vi "Validate Section ID.vi"(6 "Name":string, 8 "error in (no error)":errorcluster, 11 "Ref ID in":T1 format="%.0x") -> (0 "error out":errorcluster, 3 "Ref ID out":T1 format="%.0x")   [LabVIEW 2017, in "SLSC Switch Scripting.lvlib"]
uses:
  <vilib>/NI Veristand/Custom Device API/Custom Device Item Ref.ctl
  NationalInstruments.VeriStand.SystemDefinitionAPI
  SLSC Switch Scripting.lvlib
  <vilib>/NI VeriStand/Custom Device API/Custom Device API.lvlib
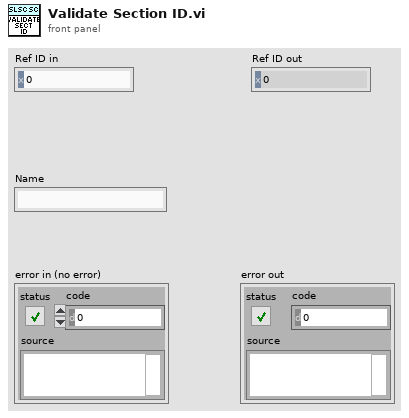
[diagram p1: front panel]
types:
  T1 = typedef "Custom Device API.lvlib/Custom Device Item Ref.ctl" = u64
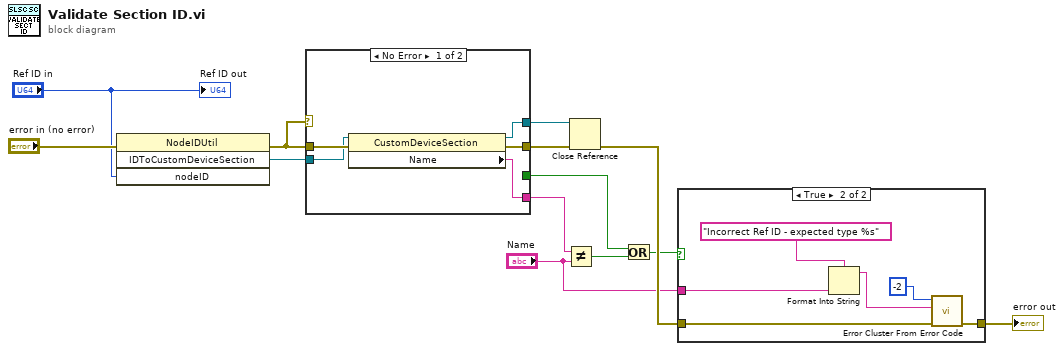
[diagram p0: block diagram]
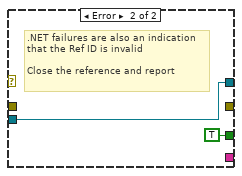
[diagram p2: hidden frame]
diagram:
  n1 = invoke class="NodeIDUtil" method="IDToCustomDeviceSection"(error in="error in (no error)", "nodeID"="Ref ID in") -> (error out=w4:errorcluster, "IDToCustomDeviceSection"=w10:refnum<k24>)  [unwired: 2 in, 2 out]
  n2 = case shown="No Error" w4 {
    tunnel: [w18 _] -> w13
    tunnel: [w17 _] -> w12
    tunnel: [w16 w20] -> w11
    tunnel: w4 -> [w15 _]
    tunnel: w10 -> [w14 w20]
    tunnel: [_ TRUE] -> w2
    frame No Error {
      n3 = property class="CustomDeviceSection"(reference=w14, error in=w15) -> (reference out=w16:refnum<k24>, error out=w17:errorcluster, "Name"=w18:string)
    }
    frame Error {
      # ".NET failures are also an indication\nthat the Ref ID is invalid\n\nClose the reference and report"
    }
  }
  n4 = Not Equal?(x=w13, y="Name") -> (x != y?=w1:bool)
  n5 = Close Reference(reference=w11, error in (no error)=w12) -> (error out=w8:errorcluster)
  n6 = Or(x=w2, y=w1) -> (x .or. y?=w3:bool)
  n7 = case shown="True" w3 {
    tunnel: w8 -> [w21 w26]
    tunnel: [w21 w25] -> w7
    tunnel: "Name" -> [_ w23]
    frame False {
    }
    frame True {
      n8 = Format Into String(format string="Incorrect Ref ID - expected type %s" ("error message (\"\")"), w23) -> (resulting string=w22:string)  [unwired: 2 in, 1 out]
      n9 = call <vilib>:"Error Cluster From Error Code.vi"("error in (no error)"=w26, "error message (\"\")"=w22, "error code (0)"=-2) -> ("error out"=w25:errorcluster)  [unwired: 6 in]
    }
  }
  "error out" <- w7
  "Ref ID out" <- "Ref ID in"
